vi "Close.vi"(8 "error in (no error)":errorcluster, 11 "TelemetryDebug in":refnum<class "TelemetryDebug.lvclass">) -> (0 "error out":errorcluster)   [LabVIEW 2020, in "VectoTools.lvlib" / "TelemetryDebug.lvclass"]
uses:
  TelemetryDebug.lvclass
  TelemetryDebug.lvclass/TelemetryDebug.ctl
  Vecto/RemoteDataService/RemoteDataService.lvclass
  Vecto/ChannelService/ChannelService.lvclass
  Vecto/DiscoveryService/DiscoveryService.lvclass
  Vecto/SequenceCountService/SequenceCountService.lvclass
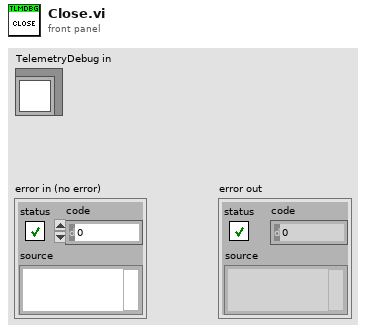
[diagram p1: front panel]
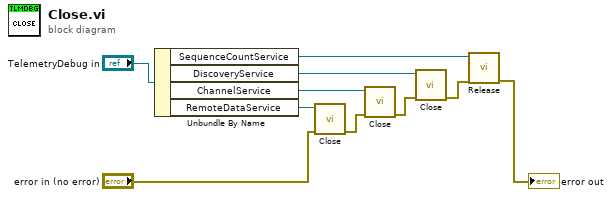
[diagram p0: block diagram]
diagram:
  n1 = Unbundle By Name("TelemetryDebug in") -> ("SequenceCountService"=w4:refnum<class "SequenceCountService.lvclass">, "DiscoveryService"=w6:refnum<class "DiscoveryService.lvclass">, "ChannelService"=w8:refnum<class "ChannelService.lvclass">, "RemoteDataService"=w9:refnum<class "RemoteDataService.lvclass">)
  n2 = call "Close.vi"("error in (no error)"="error in (no error)", "RemoteDataService in"=w9) -> ("error out"=w7:errorcluster)  [unwired: 9 in]
  n3 = call "Close.vi"("error in (no error)"=w7, "ChannelService in"=w8) -> ("error out"=w5:errorcluster)  [unwired: 9 in]
  n4 = call "Close.vi"("error in (no error)"=w5, "DiscoveryService in"=w6) -> ("error out"=w3:errorcluster)  [unwired: 9 in]
  n5 = call "Release.vi"("error in (no error)"=w3, "SequenceCountService in"=w4) -> ("error out"=→"error out":errorcluster)  [unwired: 9 in]
